vi "Orient.vi"(8 "error in (no error)":errorcluster, 9 "Yaw":sgl, 10 "Pitch":sgl, 11 "3D Object in":refnum<class "3D Object.lvclass">) -> (0 "error out":errorcluster, 3 "3D Object out":refnum<class "3D Object.lvclass">)   [LabVIEW 2015, in "3D Object.lvclass"]
uses:
  3D Object.lvclass
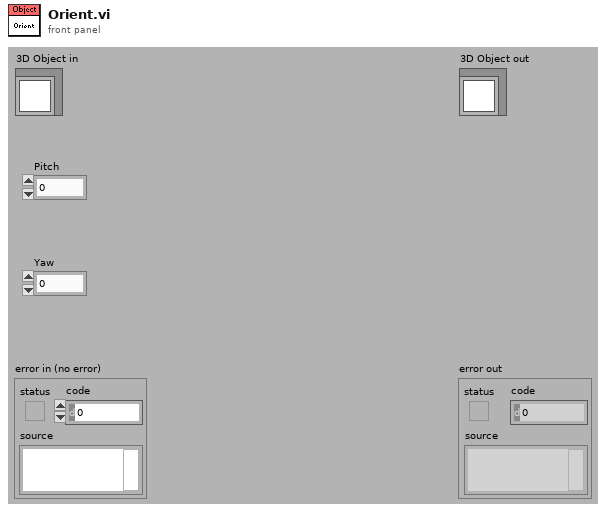
[diagram p1: front panel]
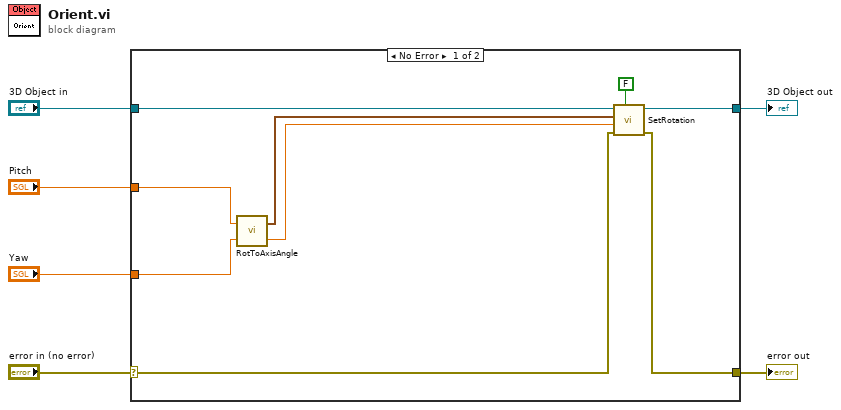
[diagram p0: block diagram]
diagram:
  n1 = case shown="No Error" "error in (no error)" {
    selector: "error in (no error)" -> [w11 w17]
    tunnel: [w15 w17] -> w5
    tunnel: [w14 w16] -> w4
    tunnel: "3D Object in" -> [w12 w16]
    tunnel: "Pitch" -> [w8 _]
    tunnel: "Yaw" -> [w7 _]
    frame No Error {
      n2 = call "RotToAxisAngle.vi"("Yaw"=w7, "Pitch"=w8) -> ("Angle"=w9:sgl, "Axis"=w10:cluster{"X":sgl, "Y":sgl, "Z":sgl})
      n3 = call "SetRotation.vi"("Relative?"=FALSE, "error in (no error)"=w11, "Angle"=w9, "Axis"=w10, "3D Object in"=w12) -> ("error out"=w15:errorcluster, "3D Object out"=w14:refnum<class "3D Object.lvclass">)  [unwired: 5 in]
    }
    frame Error {
    }
  }
  "error out" <- w5
  "3D Object out" <- w4
